vi "Disable Caching.vi"(8 "error in (no error)":errorcluster, 11 "Response in":refnum<class "Response.lvclass">) -> (0 "error out":errorcluster, 3 "Response out":refnum<class "Response.lvclass">)   [LabVIEW 2020, in "HTTP Utils.lvlib" / "Response.lvclass"]
uses:
  Response.lvclass
  Response.lvclass/Response.ctl
  Cache Directive.ctl
  HTTP Utils.lvlib
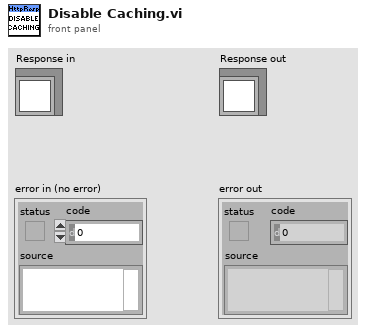
[diagram p1: front panel]
types:
  T1 = typedef "HTTP Utils.lvlib/Cache Directive.ctl" = enum16{"None (no-store)", "Always Validate (no-cache)", "Private Only (private)", "Always Allow (public)"}
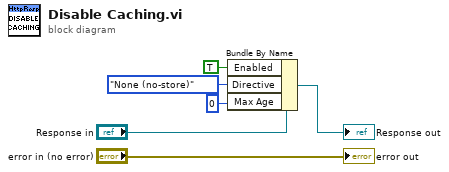
[diagram p0: block diagram]
diagram:
  n1 = Bundle By Name(cluster="Response in", "Enabled"=TRUE ("Cache Params.Enabled"), "Directive"=Cache_Directive."None (no-store)" ("Cache Params.Directive"), "Max Age"=0 ("Cache Params.Max Age")) -> (→"Response out":refnum<class "Response.lvclass">)
  "error out" <- "error in (no error)"
